vi "Auto 9.vi"(8 "Error In":errorcluster) -> (0 "Error Out":errorcluster)   [LabVIEW 2014]
uses:
  <vilib>/Rock Robotics/Network Tables/SD Read Boolean.vi
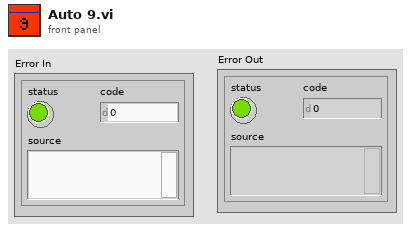
[diagram p1: front panel]
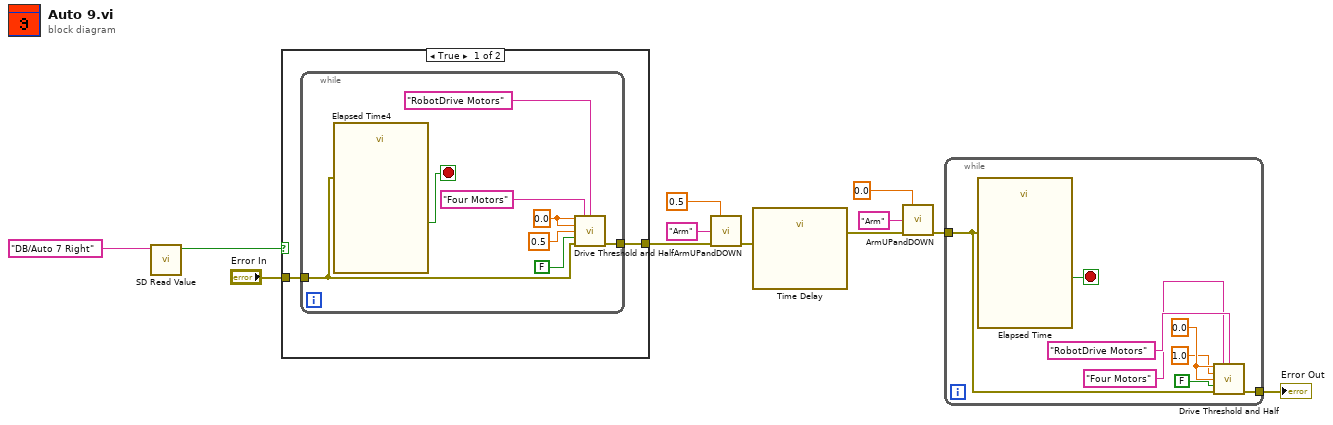
[diagram p0: block diagram]
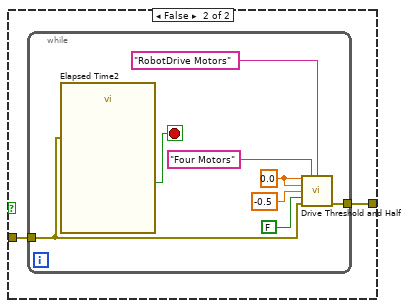
[diagram p2: hidden frame]
diagram:
  n1 = call-poly <vilib>:"SD Read Value.vi"("Name"="DB/Auto 7 Right") -> ("Boolean"=w3:bool)  [unwired: 8 in, 2 out]
  n2 = case shown="True" w3 {
    tunnel: [w14 w24] -> w1
    tunnel: "Error In" -> [w13 w23]
    frame True {
      n3 = while {
        tunnel: [w19] -> w14
        tunnel: w13 -> [w15]
        stop <- w16 stop-if-true
        w18 = 0.0 ("Arm Value")
        n4 = call "Elapsed Time4"("error in (no error)"=w15) -> ("Time has Elapsed"=w16:bool)  [unwired: 11 in, 7 out]
        n5 = call "Drive Threshold and Half.vi"("X In"=w18, "Drive refnum name"="Four Motors" ("refnum name"), "Send to DB Name"="RobotDrive Motors" ("Name"), "Y In"=w18, "R In"=0.5 ("X In"), "Speed Toggle"=FALSE ("Grabber Open/Close"), "Error In"=w15) -> ("Error Out"=w19:errorcluster)  [unwired: 8 in]
      }
    }
    frame False {
      n6 = while {
        tunnel: [w27] -> w24
        tunnel: w23 -> [w25]
        stop <- w26 stop-if-true
        w29 = 0.0 ("Arm Value")
        n7 = call "Elapsed Time2"("error in (no error)"=w25) -> ("Time has Elapsed"=w26:bool)  [unwired: 11 in, 7 out]
        n8 = call "Drive Threshold and Half.vi"("X In"=w29, "Drive refnum name"="Four Motors" ("refnum name"), "Send to DB Name"="RobotDrive Motors" ("Name"), "Y In"=w29, "R In"=-0.5 ("X In"), "Speed Toggle"=FALSE ("Grabber Open/Close"), "Error In"=w25) -> ("Error Out"=w27:errorcluster)  [unwired: 8 in]
      }
    }
  }
  n9 = call "ArmUPandDOWN.vi"("Arm Value"=0.5, "Arm"="Arm" ("refnum name"), "Error In"=w1) -> ("Error Out"=w12:errorcluster)  [unwired: 12 in]
  n10 = call "Time Delay"("error in (no error)"=w12) -> ("error out"=w7:errorcluster)  [unwired: 10 in]
  n11 = call "ArmUPandDOWN.vi"("Arm Value"=0.0, "Arm"="Arm" ("refnum name"), "Error In"=w7) -> ("Error Out"=w6:errorcluster)  [unwired: 12 in]
  n12 = while {
    tunnel: w6 -> [w33]
    tunnel: [w37] -> w5
    stop <- w34 stop-if-true
    w36 = 0.0 ("Arm Value")
    n13 = call "Elapsed Time"("error in (no error)"=w33) -> ("Time has Elapsed"=w34:bool)  [unwired: 11 in, 7 out]
    n14 = call "Drive Threshold and Half.vi"("X In"=w36, "Drive refnum name"="Four Motors" ("refnum name"), "Send to DB Name"="RobotDrive Motors" ("Name"), "Y In"=1.0 ("X In"), "R In"=w36, "Speed Toggle"=FALSE ("Grabber Open/Close"), "Error In"=w33) -> ("Error Out"=w37:errorcluster)  [unwired: 8 in]
  }
  "Error Out" <- w5
